vi "Analog_input_ch1_Continuous_DataLogger.vi"() -> ()   [LabVIEW 2019]
uses:
  <vilib>/Waveform/WDTOps.llb/WDT Append Waveforms DBL.vi
  <vilib>/Waveform/WDTFileIO.llb/Export Waveform To Spreadsheet File.vi
panel:
  out "Waveform Chart":waveform(dbl)(graph)
  in  "stop":bool
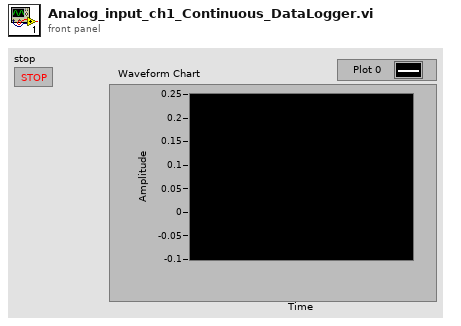
[diagram p1: front panel]
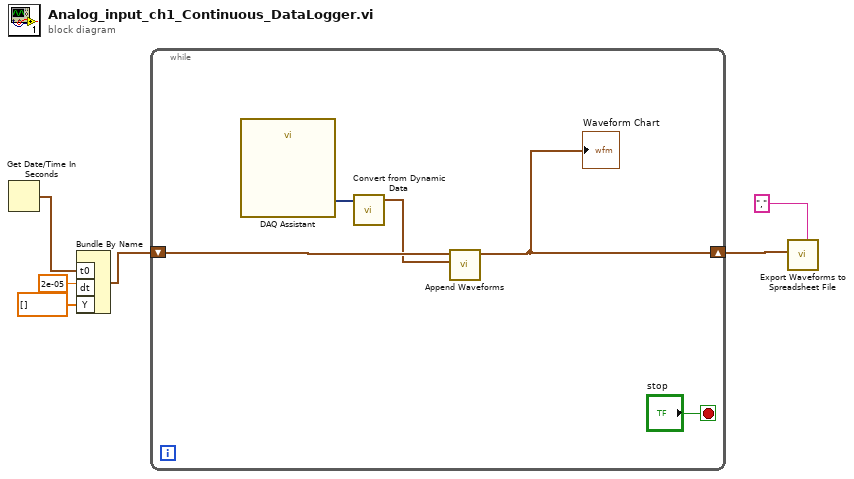
[diagram p0: block diagram]
diagram:
  n1 = Get Date/Time In Seconds() -> (seconds since 1Jan1904=w5:timestamp)
  n2 = Bundle By Name("t0"=w5, "dt"=2e-05, "Y"=dbl[] []) -> (w4:waveform(dbl))  [unwired: 1 in]
  n3 = while {
    shift-right: [w7] -> w2
    shift-left: w4 -> [w10]
    stop <- "stop" stop-if-true
    n4 = call "DAQ Assistant"() -> ("data"=w11:dynamicdata)  [unwired: 17 in, 2 out]
    n5 = call "Convert from Dynamic Data"("Dynamic Data Type"=w11) -> ("Waveform"=w9:waveform(dbl))  [unwired: 3 in]
    n6 = call-poly <vilib>:"Append Waveforms.vi"("waveform B"=w9, "waveform A"=w10) -> ("waveform out"=w7:waveform(dbl))  [unwired: 8 in, 1 out]
    "Waveform Chart" <- w7
  }
  n7 = call-poly <vilib>:"Export Waveforms to Spreadsheet File.vi"("delimiter (Tab)"=",", "waveform"=w2) -> ()  [unwired: 8 in, 2 out]
